vi "Main.vi"(10 "Number of socket":i32, 11 "Module Admin":refnum<class "Delacor_lib_QMH_Cloneable Module Admin.lvclass">) -> ()   [LabVIEW 2019, in "Test Unit.lvlib"]
doc: "This template is based off of the Queued Message Handler design pattern and the Queued Message Handler project template that ships with LabVIEW.\n\nThe main difference is that the queue is private to this module and communication between modules is performed via Broadcast and Request events.\n\nRequest events are wrapped in public API methods and are handled in the Event Handling Loop (EHL) of this VI. Any module can register for Broadcast events sent by this module. The EHL generates messages based on user interface actions.\n\nThe Message Handling Loop (MHL) processes messages generated by the EHL, or by other messages. The messages are string values, so new messages can be added easily to the Message Cases case structure in the MHL. Each message cluster can also provide an optional value for Message Data, which is a variant that can be converted to whatever message-specific data is required.\n_____\nBased on DQMH Project Template 7.0.1.1316."
uses:
  Test Unit.lvlib
  <vilib>/Delacor/Delacor QMH/Libraries/Cloneable Module Admin_class/Delacor_lib_QMH_Cloneable Module Admin.lvclass
  C:/Program Files (x86)/National Instruments/LabVIEW 2019/vi.lib/Delacor/Delacor QMH/Libraries/Module Admin_class/Delacor_lib_QMH_Module Admin.lvclass
  System.Windows.Forms
  <vilib>/Delacor/Delacor QMH/Libraries/Cloneable Module Admin_class/Delacor_lib_QMH_Cloneable Module Admin.lvclass/Delacor_lib_QMH_Cloneable Module Admin.ctl
  Module Data--cluster.ctl
  UUT Result.ctl
  <vilib>/Test Bench Framework/Test Executive.lvlibp/TestEngine/TestEngine/TestEngine/Typedefs/Report General.ctl
  <vilib>/Delacor/Delacor QMH/Libraries/Message Queue_class/Delacor_lib_QMH_Message Queue.lvclass/Delacor_lib_QMH_Message Queue.ctl
  Full User Interface/Send User Message Argument--cluster.ctl
  Stop Argument--cluster.ctl
  <vilib>/Delacor/Delacor QMH/Libraries/Module Admin_class/Delacor_lib_QMH_Module Admin.lvclass/Delacor_lib_QMH_Module Admin.ctl
  TitleWindows Argument--cluster.ctl
  Cofiguration Argument--cluster.ctl
  <vilib>/Test Bench Framework/Test Executive.lvlibp/TestEngine/TestEngine/TestEngine/Typedefs/TestEngine Cofiguration.ctl
  <vilib>/Test Bench Framework/Test Executive.lvlibp/TestEngine/TestEngine/TestEngine/Typedefs/Local Report Configuration.ctl
  <vilib>/Test Bench Framework/Test Executive.lvlibp/TestEngine/TestEngine/TestEngine/Report Format.ctl
  <vilib>/Test Bench Framework/Test Executive.lvlibp/TestEngine/TestEngine/TestEngine/Typedefs/Database Configuration.ctl
  Load Sequence Argument--cluster.ctl
  Write SN Argument--cluster.ctl
  UUT Test Argument--cluster.ctl
  UUTs Test Argument--cluster.ctl
  Terminate Test Argument--cluster.ctl
  Set Variable Argument--cluster.ctl
  Get Variable Argument--cluster.ctl
  Get Variable (Reply Payload)--cluster.ctl
  <vilib>/Delacor/Delacor QMH/Libraries/Message Queue_class/Delacor_lib_QMH_Enqueue Message (Single).vi
  <vilib>/Delacor/Delacor QMH/Libraries/Cloneable Module Admin_class/Delacor_lib_QMH_Get Module ID.vi
  <vilib>/Delacor/Delacor QMH/Libraries/Module Admin_class/Delacor_lib_QMH_Get External Launch.vi
  ffe5634f-0fac-49bb-99a4-0389974cdd12.vi
  <vilib>/Delacor/Delacor QMH/Libraries/Message Queue_class/Delacor_lib_QMH_Message Queue.lvclass
  <vilib>/Test Bench Framework/Test Executive(API).lvlib
  <vilib>/Test Bench Framework/Test Executive.lvlibp/TestEngine/TestEngine/TestEngine/Test Engine.lvclass
  Full User Interface/Full User Interface.lvlib
panel:
  in  "Panel":refnum<k24>(container)
  out "error out":errorcluster
  out "Status":string
  in  "Simulate EHL Error":bool
  in  "Simulate MHL Error":bool
  # "Other processes communicate with this Module via its Public API (wrappers for its Request Events).\n\nThis Module communicates with other processes via its Broadcast Events.\nAny process that wants to receive these messages can register for this module's Broadcast events."
  # "This template is for the DQMH framework. See the block diagram for more information on how to use this template."
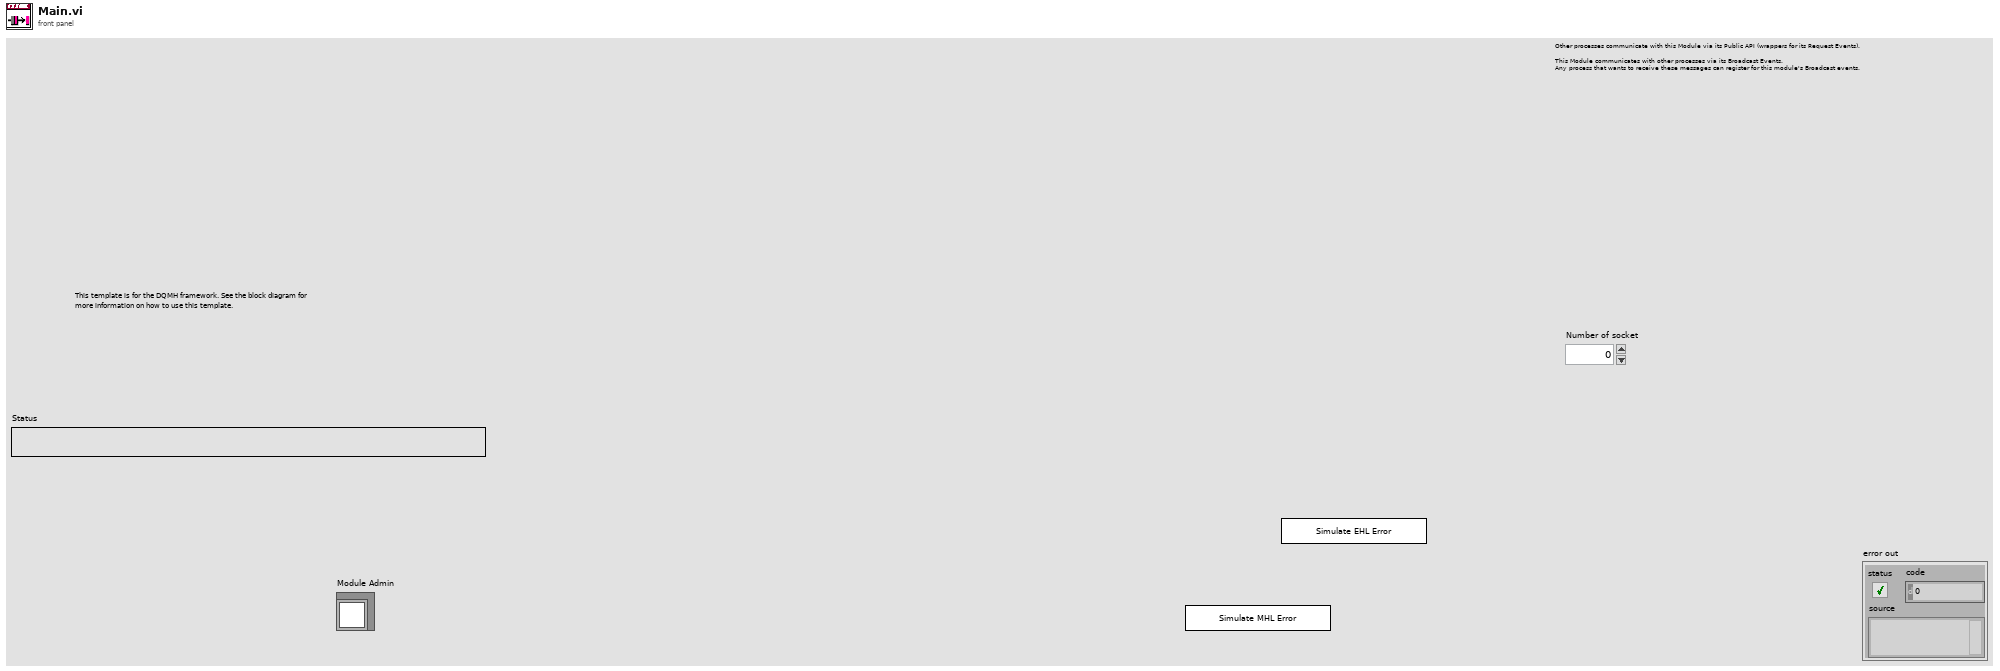
[diagram p1: front panel]
types:
  T1 = typedef "Test Unit.lvlib/Request Events--cluster.ctl" = cluster{"Stop Module":refnum<user-event>, "Show Panel":refnum<user-event>, "Hide Panel":refnum<user-event>, "Show Diagram":refnum<user-event>, "Get Module Execution Status":refnum<user-event>, "TileWindows":refnum<user-event>, "TitleWindows":refnum<user-event>, "Cofiguration":refnum<user-event>, "Load Sequence":refnum<user-event>, "Write SN":refnum<user-event>, "UUT Test":refnum<user-event>, "UUTs Test":refnum<user-event>, "Terminate Test":refnum<user-event>, "Set Variable":refnum<user-event>, "Get Variable":refnum<user-event>}
  T2 = cluster{"Event Registration Refnum":refnum<event-registration>, "Event Registration Refnum":refnum<event-registration>}
  T3 = typedef "Test Unit.lvlib/Module Data--cluster.ctl" = cluster{"Status":string, "exit":refnum<user-event>[], "UUT Result":map{i32, refnum<user-event>}}
  T4 = typedef "Test Unit.lvlib/UUT Result.ctl" = cluster{"Station":i32, "Socket":i32, "DetailTestResult":string[][], "Report Path":path, "General":T5}
  T5 = typedef "Test Executive.lvlibp/Test Engine.lvlib/Test Engine.lvclass/Report General.ctl" = cluster{"Sequence Path":path, "Serial Number":string, "Test Date Time":timestamp, "UUT Status":string, "Faulty Item":string, "Seconds Executing":dbl}
  T6 = typedef "Full User Interface.lvlib/Send User Message Argument--cluster.ctl" = cluster{"Station ID":i32, "Socket":i32, "UserMessage":string, "MessageData":variant}
  T7 = enum32{"invalid lock state", "Not Locked", "Locked (No Password)", "Password-protected"}
  T8 = typedef "Test Unit.lvlib/Stop Argument--cluster.ctl" = cluster{"Module ID":i32, "Origin":string, "Exit via Stop Module Req?":bool, "Wait for Module to stop?":bool}
  T9 = typedef "Test Unit.lvlib/TitleWindows Argument--cluster.ctl" = cluster{"Module ID":i32, "TitleWindows":bool, "dont initi":bool}
  T10 = typedef "Test Unit.lvlib/Cofiguration Argument--cluster.ctl" = cluster{"Module ID":i32, "TestEngine Cofiguration":T11}
  T11 = typedef "Test Executive.lvlibp/Test Engine.lvlib/Test Engine.lvclass/TestEngine Cofiguration.ctl" = cluster{"Break on Failure":bool, "Automatically handle TestVI error":cluster{"Enable":bool, "Handle":enum16{"Termination test", "Ignore error"}}, "Local Report Configuration":T12, "Database Configuration":T14, "Ignore breakpoint":bool, "Filter Result":bool}
  T12 = typedef "Test Executive.lvlibp/Test Engine.lvlib/Test Engine.lvclass/Local Report Configuration.ctl" = cluster{"Report Folder Path":path, "Format":T13, "Disable":bool, "Build Date Folder?":bool}
  T13 = typedef "Test Executive.lvlibp/Test Engine.lvlib/Test Engine.lvclass/Report Format.ctl" = enum16{"Excel", "CSV(Tab)", "CSV(,)", "CSV(;)", "TEXT", "HTML"}
  T14 = typedef "Test Executive.lvlibp/Test Engine.lvlib/Test Engine.lvclass/Database Configuration.ctl" = cluster{"Connection String Expression":string, "Microsoft Data Link File":path, "Connection Type":enum16{"Use Connection String Expression", "Use Microsoft Data Link File"}, "Enable":bool}
  T15 = typedef "Test Unit.lvlib/Load Sequence Argument--cluster.ctl" = cluster{"Module ID":i32, "File Pathname":path, "Sequence":string}
  T16 = typedef "Test Unit.lvlib/Write SN Argument--cluster.ctl" = cluster{"Module ID":i32, "Socket":i32, "Serial Number":string}
  T17 = typedef "Test Unit.lvlib/UUT Test Argument--cluster.ctl" = cluster{"Module ID":i32, "Socket":i32}
  T18 = typedef "Test Unit.lvlib/UUTs Test Argument--cluster.ctl" = cluster{"Module ID":i32, "Enable Socket":bool[]}
  T19 = typedef "Test Unit.lvlib/Terminate Test Argument--cluster.ctl" = cluster{"Module ID":i32, "Abort VI":bool}
  T20 = typedef "Test Unit.lvlib/Set Variable Argument--cluster.ctl" = cluster{"Module ID":i32, "Variable":string, "Socket":i32, "Value":variant}
  T21 = typedef "Test Unit.lvlib/Get Variable Argument--cluster.ctl" = cluster{"Module ID":i32, "Socket":i32, "Variable":string, "Wait Notifier":refnum<notifier>, "wait for reply":bool}
  T22 = enum32{"Invalid", "Standard", "Closed", "Hidden", "Minimized", "Maximized"}
  T23 = typedef "Test Unit.lvlib/Get Variable (Reply Payload)--cluster.ctl" = cluster{"Module ID":i32, "Value":variant, "Variable not found?":bool, "timed out?":bool, "error":errorcluster}
  T24 = cluster{"Left":i32, "Top":i32, "Right":i32, "Bottom":i32}
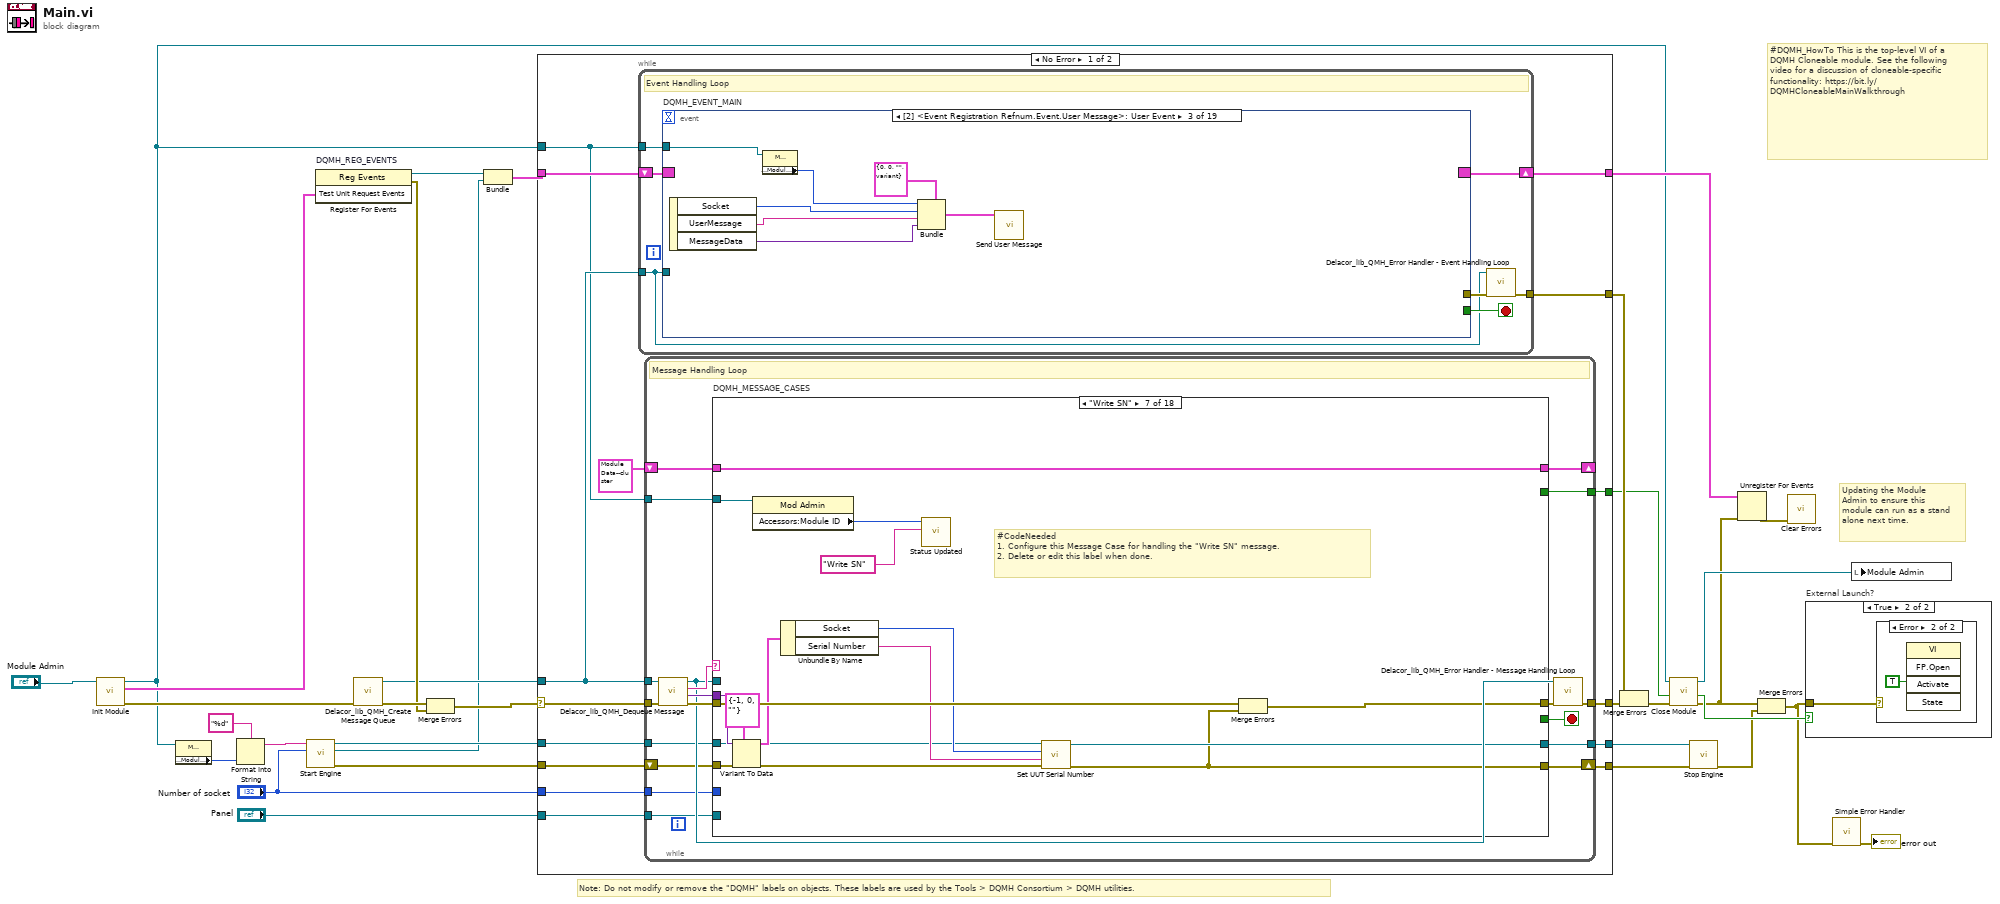
[diagram p0: block diagram]
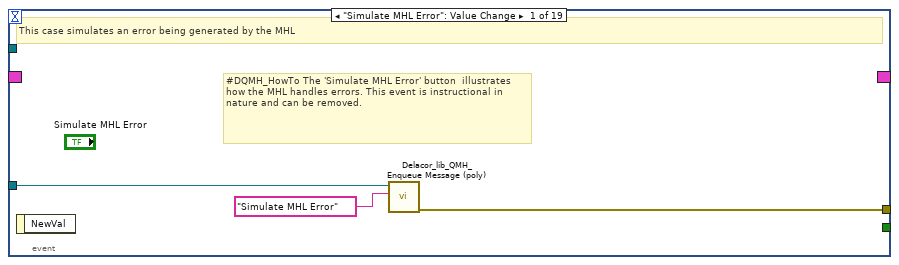
[diagram p2: hidden frame]
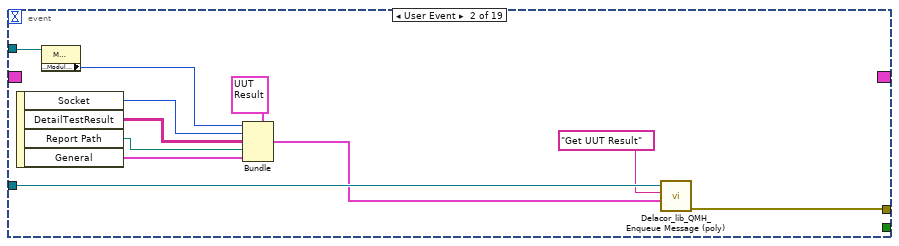
[diagram p3: hidden frame]
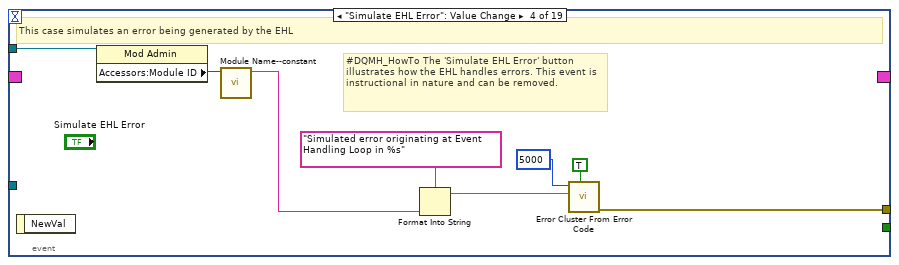
[diagram p4: hidden frame]
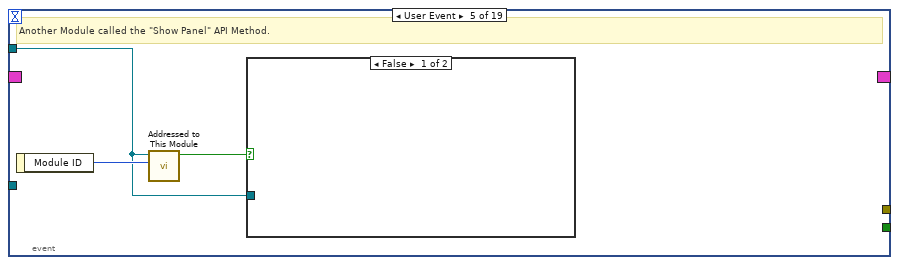
[diagram p5: hidden frame]
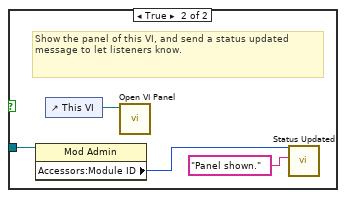
[diagram p6: hidden frame]
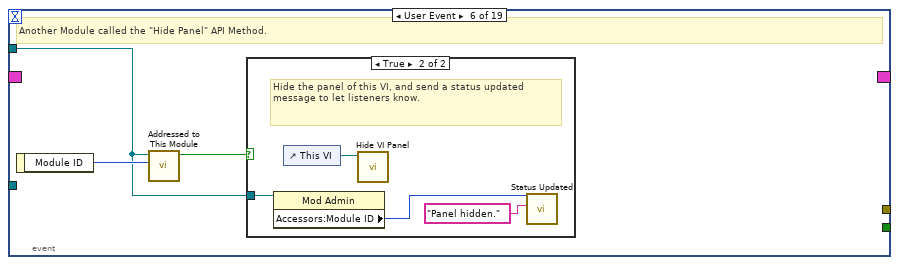
[diagram p7: hidden frame]
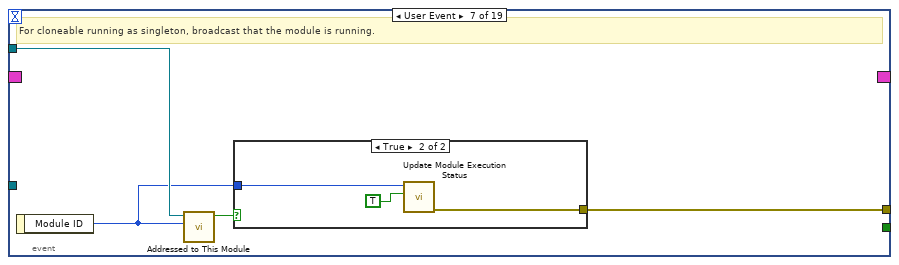
[diagram p9: hidden frame]
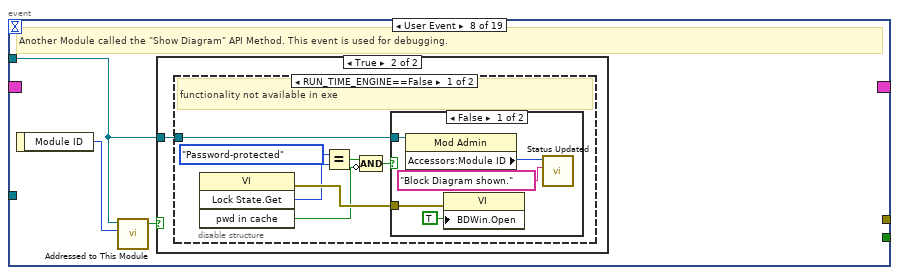
[diagram p11: hidden frame]
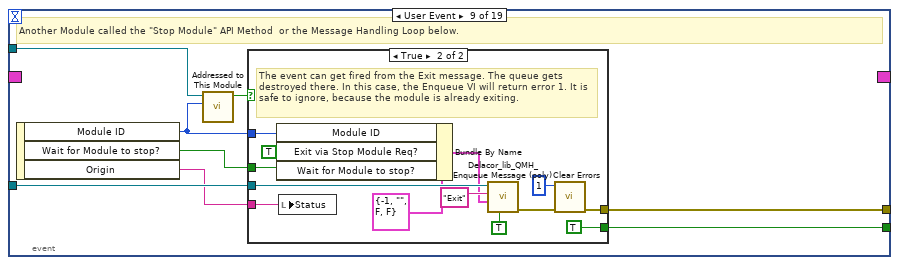
[diagram p15: hidden frame]
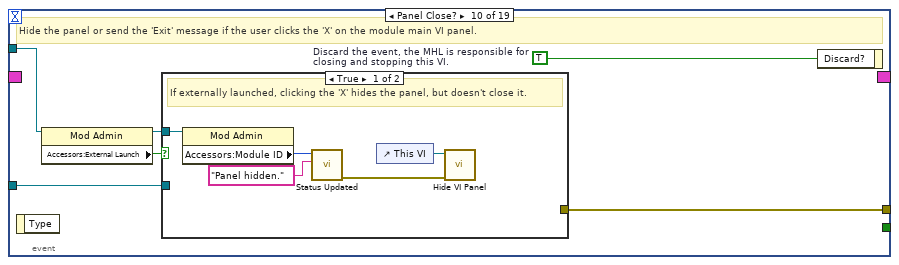
[diagram p17: hidden frame]
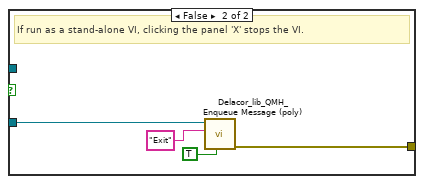
[diagram p18: hidden frame]
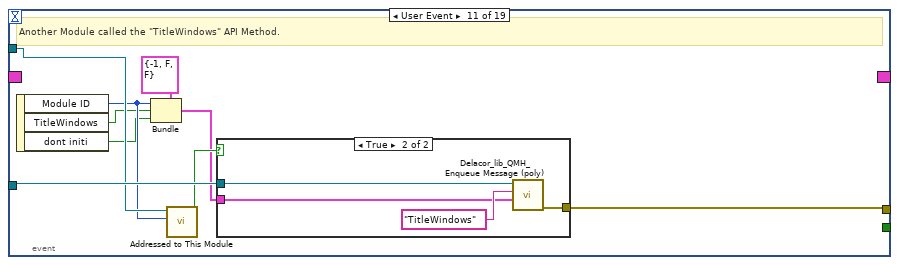
[diagram p19: hidden frame]
diagram:
  # "#DQMH_HowTo This is the top-level VI of a DQMH Cloneable module. See the following video for a discussion of cloneable-specific functionality: https://bit.ly/DQMHCloneableMainWalkthrough"
  # "Note: Do not modify or remove the \"DQMH\" labels on objects. These labels are used by the Tools > DQMH Consortium > DQMH utilities."
  # "Updating the Module Admin to ensure this module can run as a stand alone next time."
  n1 = call "Init Module.vi"("Cloneable Module Admin in"="Module Admin") -> ("error out"=w29:errorcluster, "Test Unit Request Events"=w24:T1, "Cloneable Module Admin out"=w17:refnum<class "Delacor_lib_QMH_Cloneable Module Admin.lvclass">)  [unwired: 8 in]
  n2 = property class="Mod Admin"(reference=w17) -> ("Accessors:Module ID"=w16:i32)  [unwired: 1 in, 2 out]
  n3 = Format Into String(format string="%d", w16) -> (resulting string=w14:string)  [unwired: 2 in, 1 out]
  n4 = call <vilib>:"Start Engine.vi"("Number of Socket"="Number of socket", "Process"=w14) -> ("error out"=w19:errorcluster, "Event Registration Refnum"=w3:refnum<event-registration>, "Test Executive Manage out"=w18:refnum<class "Test Executive Manage.lvclass">)  [unwired: 7 in]
  n5 = register-events "DQMH_REG_EVENTS"(w24) -> (reference out=w25:refnum<event-registration>, error out=w27:errorcluster)  [unwired: 2 in]
  n6 = call <vilib>:"Delacor_lib_QMH_Create Message Queue.vi"("error in"=w29) -> ("error out"=w28:errorcluster, "Message Queue"=w10:refnum<class "Delacor_lib_QMH_Message Queue.lvclass">)  [unwired: 9 in]
  n7 = Merge Errors(w28, w27) -> (w9:errorcluster)
  n8 = Bundle("Event Registration Refnum"=w25, "Event Registration Refnum"=w3) -> (w4:T2)  [unwired: 1 in]
  n9 = case shown="No Error" w9 {
    selector: w9 -> [w45 w611]
    tunnel: [w47 w610] -> w30
    tunnel: [w44 w609] -> w26
    tunnel: w4 -> [w42 w609]
    tunnel: w10 -> [w41 w602]
    tunnel: [w46 _] -> w31
    tunnel: w17 -> [w40 w605]
    tunnel: [w39 _] -> w21
    tunnel: w19 -> [w38 w600]
    tunnel: w18 -> [w37 w601]
    tunnel: [w36 w601] -> w13
    tunnel: [w35 w600] -> w12
    tunnel: "Number of socket" -> [w34 _]
    tunnel: "Panel" -> [w33 _]
    frame No Error {
      n10 = while {
        tunnel: w41 -> [w48]
        shift-right: [w51] -> w44
        shift-left: w42 -> [w52]
        tunnel: [w53] -> w46
        tunnel: w40 -> [w49]
        stop <- w50 stop-if-true
        # "Event Handling Loop"
        n11 = event "DQMH_EVENT_MAIN" shown="[2] <Event Registration Refnum.Event.User Message>: User Event" {
          selector: w52 -> [_ _ _ _ _ _ _ _ _ _ _ _ _ _ _ _ _ _ _]
          dyn-events: [_ _ _ _ _ _ _ _ _ _ _ _ _ _ _ _ _ _ _] -> w51
          timeout: _ -> [_ _ _ _ _ _ _ _ _ _ _ _ _ _ _ _ _ _ _]
          tunnel: [_ _ _ _ _ _ _ _ w124 _ _ _ _ _ _ _ _ _ _] -> w50
          tunnel: w48 -> [w56 w68 _ _ _ _ _ _ w127 w144 w165 w177 w190 w203 w215 w227 w239 w253 w268]
          tunnel: [w57 w66 _ w83 _ _ w101 _ w128 w147 w158 w170 w182 w195 w208 w220 w232 w244 w258] -> w54
          tunnel: w49 -> [_ w63 w75 w82 w84 w91 w99 w105 w126 w145 w163 w175 w188 w201 w213 w225 w237 w251 w266]
          event "Simulate MHL Error": Value Change {
            # "#DQMH_HowTo The 'Simulate MHL Error' button  illustrates how the MHL handles errors. This event is instructional in nature and can be removed."
            # "This case simulates an error being generated by the MHL"
            n12 = event-data() -> ()  [unwired: 1 in, 1 out]
            n13 = call-poly <vilib>:"Delacor_lib_QMH_Enqueue Message (poly).vi"("Message"="Simulate MHL Error", "Message Queue in"=w56) -> ("error out"=w57:errorcluster)  [unwired: 8 in, 1 out]
          }
          event User Event {
            n14 = event-data() -> ("Socket"=w61:i32, "DetailTestResult"=w60:string[][], "Report Path"=w59:path, "General"=w58:T5)  [unwired: 1 in]
            n15 = property class="Mod Admin"(reference=w63) -> ("Accessors:Module ID"=w62:i32)  [unwired: 1 in, 2 out]
            n16 = Bundle(cluster=T4 {"Station"=0, "Socket"=0, "DetailTestResult"=[], "Report Path"=path "", "General"={"Sequence Path"=path "", "Serial Number"="", "Test Date Time"=timestamp(0 s since 1904-01-01), "UUT Status"="", "Faulty Item"="", "Seconds Executing"=0.0}} ("output cluster"), "Station"=w62, "Socket"=w61, "DetailTestResult"=w60, "Report Path"=w59, "General"=w58) -> (w67:T4)
            n17 = call-poly <vilib>:"Delacor_lib_QMH_Enqueue Message (poly).vi"("Message Data"=w67, "Message"="Get UUT Result", "Message Queue in"=w68) -> ("error out"=w66:errorcluster)  [unwired: 7 in, 1 out]
          }
          event User Event {
            n18 = event-data() -> ("Socket"=w72:i32, "UserMessage"=w71:string, "MessageData"=w70:variant)  [unwired: 1 in]
            n19 = property class="Mod Admin"(reference=w75) -> ("Accessors:Module ID"=w73:i32)  [unwired: 1 in, 2 out]
            n20 = Bundle(cluster=T6 {"Station ID"=0, "Socket"=0, "UserMessage"="", "MessageData"=variant(cluster{"Socket":i32, "UserMessage":string, "MessageData":variant} {"Socket"=0, "UserMessage"="", "MessageData"=variant})} ("DQMH_ARG"), "Station ID"=w73, "Socket"=w72, "UserMessage"=w71, "MessageData"=w70) -> (w69:T6)
            n21 = call "Send User Message.vi"("DQMH_ARG"=w69) -> ()  [unwired: 10 in, 1 out]
          }
          event "Simulate EHL Error": Value Change {
            # "#DQMH_HowTo The 'Simulate EHL Error' button  illustrates how the EHL handles errors. This event is instructional in nature and can be removed."
            # "This case simulates an error being generated by the EHL"
            n22 = event-data() -> ()  [unwired: 1 in, 1 out]
            n23 = property on="Property Node" class="Mod Admin"(reference=w82) -> ("Accessors:Module ID"=w81:i32)  [unwired: 1 in, 2 out]
            n24 = call "Module Name--constant.vi"("Module ID"=w81) -> ("Module Name"=w76:string)  [unwired: 10 in]
            n25 = Format Into String(format string="Simulated error originating at Event Handling Loop in %s", w76) -> (resulting string=w79:string)  [unwired: 2 in, 1 out]
            n26 = call <vilib>:"Error Cluster From Error Code.vi"("show call chain? (False)"=TRUE, "error message (\"\")"=w79, "error code (0)"=5000) -> ("error out"=w83:errorcluster)  [unwired: 6 in]
          }
          event User Event {
            # "Another Module called the \"Show Panel\" API Method."
            n27 = event-data() -> ("Module ID"=w85:i32)  [unwired: 1 in]
            n28 = call "Addressed to This Module.vi"("Module ID from Argument"=w85, "Module Admin"=w84) -> ("Addressed to this instance?"=w86:bool)  [unwired: 8 in, 1 out]
            n29 = case shown="False" w86 {
              tunnel: w84 -> [_ w88]
              frame False {
              }
              frame True {
                # "Show the panel of this VI, and send a status updated message to let listeners know."
                n30 = property on="Property Node" class="Mod Admin"(reference=w88) -> ("Accessors:Module ID"=w87:i32)  [unwired: 1 in, 2 out]
                n31 = control-ref of="This VI"() -> (w90:refnum<vi>)
                n32 = call "Open VI Panel.vi"("VI"=w90) -> ()  [unwired: 10 in, 1 out]
                n33 = call "Status Updated.vi"("Status"="Panel shown." ("format string"), "Module ID"=w87) -> ()  [unwired: 9 in, 1 out]
              }
            }
          }
          event User Event {
            # "Another Module called the \"Hide Panel\" API Method."
            n34 = event-data() -> ("Module ID"=w92:i32)  [unwired: 1 in]
            n35 = call "Addressed to This Module.vi"("Module ID from Argument"=w92, "Module Admin"=w91) -> ("Addressed to this instance?"=w93:bool)  [unwired: 8 in, 1 out]
            n36 = case shown="True" w93 {
              tunnel: w91 -> [_ w95]
              frame False {
              }
              frame True {
                # "Hide the panel of this VI, and send a status updated message to let listeners know."
                n37 = property on="Property Node" class="Mod Admin"(reference=w95) -> ("Accessors:Module ID"=w94:i32)  [unwired: 1 in, 2 out]
                n38 = control-ref of="This VI"() -> (w97:refnum<vi>)
                n39 = call "Hide VI Panel.vi"("VI"=w97) -> ()  [unwired: 10 in, 1 out]
                n40 = call "Status Updated.vi"("Status"="Panel hidden." ("format string"), "Module ID"=w94) -> ()  [unwired: 9 in, 1 out]
              }
            }
          }
          event User Event {
            # "For cloneable running as singleton, broadcast that the module is running."
            n41 = event-data() -> ("Module ID"=w98:i32)  [unwired: 1 in]
            n42 = call "Addressed to This Module.vi"("Module ID from Argument"=w98, "Module Admin"=w99) -> ("Addressed to this instance?"=w100:bool)  [unwired: 8 in, 1 out]
            n43 = case shown="True" w100 {
              tunnel: [_ w104] -> w101
              tunnel: w98 -> [_ w103]
              frame False {
              }
              frame True {
                n44 = call "Update Module Execution Status.vi"("Running?"=TRUE, "Module ID"=w103) -> ("error out"=w104:errorcluster)  [unwired: 9 in]
              }
            }
          }
          event User Event {
            # "Another Module called the \"Show Diagram\" API Method. This event is used for debugging."
            n45 = event-data() -> ("Module ID"=w106:i32)  [unwired: 1 in]
            n46 = call "Addressed to This Module.vi"("Module ID from Argument"=w106, "Module Admin"=w105) -> ("Addressed to this instance?"=w107:bool)  [unwired: 8 in, 1 out]
            n47 = case shown="True" w107 {
              tunnel: w105 -> [_ w108]
              frame False {
              }
              frame True {
                n48 = disable-structure shown="RUN_TIME_ENGINE==False" {
                  disable-tunnel: w108 -> [w109 _]
                  frame condition #0 (active) {
                    # "functionality not available in exe"
                    n49 = invoke on="Invoke Node" class="VI" method="Lock State.Get"() -> (error out=w115:errorcluster, "Get Lock State"=w114:T7, "pwd in cache"=w111:bool)  [unwired: 4 in, 1 out]
                    n50 = Equal?(x=T7."Password-protected", y=w114) -> (x = y?=w112:bool)
                    n51 = Compound Arithmetic op=AND(w112, invert w111) -> (w110:bool)
                    n52 = case shown="False" w110 {
                      tunnel: w115 -> [w120 _]
                      tunnel: w109 -> [w117 _]
                      frame False {
                        n53 = property on="Property Node" class="Mod Admin"(reference=w117) -> ("Accessors:Module ID"=w116:i32)  [unwired: 1 in, 2 out]
                        n54 = property on="Property Node" class="VI"(error in=w120, "BDWin.Open"=TRUE ("Block Diagram Window:Open")) -> ()  [unwired: 1 in, 2 out]
                        n55 = call "Status Updated.vi"("Status"="Block Diagram shown." ("format string"), "Module ID"=w116) -> ()  [unwired: 9 in, 1 out]
                      }
                      frame True {
                        # "Password-protected VI, and the password is not in the cache. Do not show the diagram."
                      }
                    }
                  }
                  frame condition #1 {
                  }
                }
              }
            }
          }
          event User Event {
            # "Another Module called the \"Stop Module\" API Method  or the Message Handling Loop below."
            n56 = event-data() -> ("Module ID"=w122:i32, "Wait for Module to stop?"=w123:bool, "Origin"=w121:string)  [unwired: 1 in]
            n57 = call "Addressed to This Module.vi"("Module ID from Argument"=w122, "Module Admin"=w126) -> ("Addressed to this instance?"=w125:bool)  [unwired: 8 in, 1 out]
            n58 = case shown="True" w125 {
              tunnel: [_ w140] -> w128
              tunnel: w127 -> [_ w136]
              tunnel: [_ TRUE] -> w124
              tunnel: w123 -> [_ w131]
              tunnel: w122 -> [_ w133]
              tunnel: w121 -> [_ w129]
              frame False {
              }
              frame True {
                # "The event can get fired from the Exit message. The queue gets destroyed there. In this case, the Enqueue VI will return error 1. It is safe to ignore, because the module is already exiting."
                n59 = Bundle By Name(cluster=T8 {"Module ID"=-1, "Origin"="", "Exit via Stop Module Req?"=FALSE, "Wait for Module to stop?"=FALSE} ("Stop Argument"), "Module ID"=w133, "Exit via Stop Module Req?"=TRUE, "Wait for Module to stop?"=w131) -> (w130:T8)
                n60 = local write "Status"(w129) -> ()
                n61 = call-poly <vilib>:"Delacor_lib_QMH_Enqueue Message (poly).vi"("Priority Message? (F)"=TRUE, "Message Data"=w130, "Message"="Exit", "Message Queue in"=w136) -> ("error out"=w141:errorcluster)  [unwired: 6 in, 1 out]
                n62 = call <vilib>:"Clear Errors.vi"("error in (no error)"=w141, "specific error code to clear (0: all)"=1) -> ("error out"=w140:errorcluster)  [unwired: 4 in, 1 out]
              }
            }
          }
          event Panel Close? {
            w146 = TRUE  # Discard the event, the MHL is responsible for closing and stopping this VI.
            # "Hide the panel or send the 'Exit' message if the user clicks the 'X' on the module main VI panel."
            n63 = event-data() -> ()  [unwired: 1 in, 1 out]
            n64 = property on="Property Node" class="Mod Admin"(reference=w145) -> (reference out=w142:refnum<class "Delacor_lib_QMH_Cloneable Module Admin.lvclass">, "Accessors:External Launch"=w143:bool)  [unwired: 1 in, 1 out]
            n65 = case shown="True" w143 {
              tunnel: w144 -> [_ w155]
              tunnel: [_ w156] -> w147
              tunnel: w142 -> [w150 _]
              frame True {
                # "If externally launched, clicking the 'X' hides the panel, but doesn't close it."
                n66 = property on="Property Node" class="Mod Admin"(reference=w150) -> ("Accessors:Module ID"=w149:i32)  [unwired: 1 in, 2 out]
                n67 = call "Status Updated.vi"("Status"="Panel hidden." ("format string"), "Module ID"=w149) -> ("error out"=w148:errorcluster)  [unwired: 9 in]
                n68 = control-ref of="This VI"() -> (w152:refnum<vi>)
                n69 = call "Hide VI Panel.vi"("error in"=w148, "VI"=w152) -> ()  [unwired: 9 in, 1 out]
              }
              frame False {
                # "If run as a stand-alone VI, clicking the panel 'X' stops the VI."
                n70 = call-poly <vilib>:"Delacor_lib_QMH_Enqueue Message (poly).vi"("Priority Message? (F)"=TRUE, "Message"="Exit", "Message Queue in"=w155) -> ("error out"=w156:errorcluster)  [unwired: 7 in, 1 out]
              }
            }
            n71 = event-data ("Event Filter Node")("Discard?"=w146) -> ()  [unwired: 1 in, 1 out]
          }
          event User Event {
            # "Another Module called the \"TitleWindows\" API Method."
            n72 = event-data() -> ("Module ID"=w160:i32, "TitleWindows"=w159:bool, "dont initi"=w157:bool)  [unwired: 1 in]
            n73 = Bundle(cluster=T9 {"Module ID"=-1, "TitleWindows"=FALSE, "dont initi"=FALSE} ("TitleWindows Argument"), "Module ID"=w160, "TitleWindows"=w159, "dont initi"=w157) -> (w161:T9)
            n74 = call "Addressed to This Module.vi"("Module ID from Argument"=w160, "Module Admin"=w163) -> ("Addressed to this instance?"=w164:bool)  [unwired: 8 in, 1 out]
            n75 = case shown="True" w164 {
              tunnel: w165 -> [_ w169]
              tunnel: w161 -> [_ w167]
              tunnel: [_ w166] -> w158
              frame False {
              }
              frame True {
                n76 = call-poly <vilib>:"Delacor_lib_QMH_Enqueue Message (poly).vi"("Message Data"=w167, "Message"="TitleWindows", "Message Queue in"=w169) -> ("error out"=w166:errorcluster)  [unwired: 7 in, 1 out]
              }
            }
          }
          event User Event {
            # "Another Module called the \"Cofiguration\" API Method."
            n77 = event-data() -> ("Module ID"=w172:i32, "TestEngine Cofiguration"=w171:T11)  [unwired: 1 in]
            n78 = Bundle(cluster=T10 {"Module ID"=-1, "TestEngine Cofiguration"={"Break on Failure"=FALSE, "Automatically handle TestVI error"={"Enable"=FALSE, "Handle"=enum."Termination test"}, "Local Report Configuration"={"Report Folder Path"=path "", "Format"=enum."Excel", "Disable"=FALSE, "Build Date Folder?"=FALSE}, "Database Configuration"={"Connection String Expression"="", "Microsoft Data Link File"=path "", "Connection Type"=enum."Use Connection String Expression", "Enable"=FALSE}, "Ignore breakpoint"=FALSE, "Filter Result"=FALSE}} ("Cofiguration Argument"), "Module ID"=w172, "TestEngine Cofiguration"=w171) -> (w173:T10)
            n79 = call "Addressed to This Module.vi"("Module ID from Argument"=w172, "Module Admin"=w175) -> ("Addressed to this instance?"=w176:bool)  [unwired: 8 in, 1 out]
            n80 = case shown="True" w176 {
              tunnel: w177 -> [_ w181]
              tunnel: w173 -> [_ w179]
              tunnel: [_ w178] -> w170
              frame False {
              }
              frame True {
                n81 = call-poly <vilib>:"Delacor_lib_QMH_Enqueue Message (poly).vi"("Message Data"=w179, "Message"="Cofiguration", "Message Queue in"=w181) -> ("error out"=w178:errorcluster)  [unwired: 7 in, 1 out]
              }
            }
          }
          event User Event {
            # "Another Module called the \"Load Sequence\" API Method."
            n82 = event-data() -> ("Module ID"=w185:i32, "File Pathname"=w184:path, "Sequence"=w183:string)  [unwired: 1 in]
            n83 = Bundle(cluster=T15 {"Module ID"=-1, "File Pathname"=path "", "Sequence"="Main_Sequence"} ("Load Sequence Argument"), "Module ID"=w185, "File Pathname"=w184, "Sequence"=w183) -> (w186:T15)
            n84 = call "Addressed to This Module.vi"("Module ID from Argument"=w185, "Module Admin"=w188) -> ("Addressed to this instance?"=w189:bool)  [unwired: 8 in, 1 out]
            n85 = case shown="True" w189 {
              tunnel: w190 -> [_ w194]
              tunnel: w186 -> [_ w192]
              tunnel: [_ w191] -> w182
              frame False {
              }
              frame True {
                n86 = call-poly <vilib>:"Delacor_lib_QMH_Enqueue Message (poly).vi"("Message Data"=w192, "Message"="Load Sequence", "Message Queue in"=w194) -> ("error out"=w191:errorcluster)  [unwired: 7 in, 1 out]
              }
            }
          }
          event User Event {
            # "Another Module called the \"Write SN\" API Method."
            n87 = event-data() -> ("Module ID"=w198:i32, "Socket"=w197:i32, "Serial Number"=w196:string)  [unwired: 1 in]
            n88 = Bundle(cluster=T16 {"Module ID"=-1, "Socket"=0, "Serial Number"=""} ("Write SN Argument"), "Module ID"=w198, "Socket"=w197, "Serial Number"=w196) -> (w199:T16)
            n89 = call "Addressed to This Module.vi"("Module ID from Argument"=w198, "Module Admin"=w201) -> ("Addressed to this instance?"=w202:bool)  [unwired: 8 in, 1 out]
            n90 = case shown="True" w202 {
              tunnel: w203 -> [_ w207]
              tunnel: w199 -> [_ w205]
              tunnel: [_ w204] -> w195
              frame False {
              }
              frame True {
                n91 = call-poly <vilib>:"Delacor_lib_QMH_Enqueue Message (poly).vi"("Message Data"=w205, "Message"="Write SN", "Message Queue in"=w207) -> ("error out"=w204:errorcluster)  [unwired: 7 in, 1 out]
              }
            }
          }
          event User Event {
            # "Another Module called the \"UUT Test\" API Method."
            n92 = event-data() -> ("Module ID"=w210:i32, "Socket"=w209:i32)  [unwired: 1 in]
            n93 = Bundle(cluster=T17 {"Module ID"=-1, "Socket"=0} ("UUT Test Argument"), "Module ID"=w210, "Socket"=w209) -> (w211:T17)
            n94 = call "Addressed to This Module.vi"("Module ID from Argument"=w210, "Module Admin"=w213) -> ("Addressed to this instance?"=w214:bool)  [unwired: 8 in, 1 out]
            n95 = case shown="True" w214 {
              tunnel: w215 -> [_ w219]
              tunnel: w211 -> [_ w217]
              tunnel: [_ w216] -> w208
              frame False {
              }
              frame True {
                n96 = call-poly <vilib>:"Delacor_lib_QMH_Enqueue Message (poly).vi"("Message Data"=w217, "Message"="UUT Test", "Message Queue in"=w219) -> ("error out"=w216:errorcluster)  [unwired: 7 in, 1 out]
              }
            }
          }
          event User Event {
            # "Another Module called the \"UUTs Test\" API Method."
            n97 = event-data() -> ("Module ID"=w222:i32, "Enable Socket"=w221:bool[])  [unwired: 1 in]
            n98 = Bundle(cluster=T18 {"Module ID"=-1, "Enable Socket"=[]} ("UUTs Test Argument"), "Module ID"=w222, "Enable Socket"=w221) -> (w223:T18)
            n99 = call "Addressed to This Module.vi"("Module ID from Argument"=w222, "Module Admin"=w225) -> ("Addressed to this instance?"=w226:bool)  [unwired: 8 in, 1 out]
            n100 = case shown="True" w226 {
              tunnel: w227 -> [_ w231]
              tunnel: w223 -> [_ w229]
              tunnel: [_ w228] -> w220
              frame False {
              }
              frame True {
                n101 = call-poly <vilib>:"Delacor_lib_QMH_Enqueue Message (poly).vi"("Message Data"=w229, "Message"="UUTs Test", "Message Queue in"=w231) -> ("error out"=w228:errorcluster)  [unwired: 7 in, 1 out]
              }
            }
          }
          event User Event {
            # "Another Module called the \"Terminate Test\" API Method."
            n102 = event-data() -> ("Module ID"=w234:i32, "Abort VI"=w233:bool)  [unwired: 1 in]
            n103 = Bundle(cluster=T19 {"Module ID"=-1, "Abort VI"=FALSE} ("Terminate Test Argument"), "Module ID"=w234, "Abort VI"=w233) -> (w235:T19)
            n104 = call "Addressed to This Module.vi"("Module ID from Argument"=w234, "Module Admin"=w237) -> ("Addressed to this instance?"=w238:bool)  [unwired: 8 in, 1 out]
            n105 = case shown="True" w238 {
              tunnel: w239 -> [_ w243]
              tunnel: w235 -> [_ w241]
              tunnel: [_ w240] -> w232
              frame False {
              }
              frame True {
                n106 = call-poly <vilib>:"Delacor_lib_QMH_Enqueue Message (poly).vi"("Message Data"=w241, "Message"="Terminate Test", "Message Queue in"=w243) -> ("error out"=w240:errorcluster)  [unwired: 7 in, 1 out]
              }
            }
          }
          event User Event {
            # "Another Module called the \"Set Variable\" API Method."
            n107 = event-data() -> ("Module ID"=w248:i32, "Variable"=w247:string, "Socket"=w246:i32, "Value"=w245:variant)  [unwired: 1 in]
            n108 = Bundle(cluster=T20 {"Module ID"=-1, "Variable"="", "Socket"=0, "Value"=variant} ("Set Variable Argument"), "Module ID"=w248, "Variable"=w247, "Socket"=w246, "Value"=w245) -> (w249:T20)
            n109 = call "Addressed to This Module.vi"("Module ID from Argument"=w248, "Module Admin"=w251) -> ("Addressed to this instance?"=w252:bool)  [unwired: 8 in, 1 out]
            n110 = case shown="True" w252 {
              tunnel: w253 -> [_ w257]
              tunnel: w249 -> [_ w255]
              tunnel: [_ w254] -> w244
              frame False {
              }
              frame True {
                n111 = call-poly <vilib>:"Delacor_lib_QMH_Enqueue Message (poly).vi"("Message Data"=w255, "Message"="Set Variable", "Message Queue in"=w257) -> ("error out"=w254:errorcluster)  [unwired: 7 in, 1 out]
              }
            }
          }
          event User Event {
            # "Another Module called the \"Get Variable\" API Method."
            n112 = event-data() -> ("Module ID"=w263:i32, "Socket"=w262:i32, "Variable"=w261:string, "Wait Notifier"=w260:refnum<notifier>, "wait for reply"=w259:bool)  [unwired: 1 in]
            n113 = Bundle(cluster=T21 {"Module ID"=-1, "Socket"=0, "Variable"="", "Wait Notifier"=refnum, "wait for reply"=FALSE} ("Get Variable Argument"), "Module ID"=w263, "Socket"=w262, "Variable"=w261, "Wait Notifier"=w260, "wait for reply"=w259) -> (w264:T21)
            n114 = call "Addressed to This Module.vi"("Module ID from Argument"=w263, "Module Admin"=w266) -> ("Addressed to this instance?"=w267:bool)  [unwired: 8 in, 1 out]
            n115 = case shown="True" w267 {
              tunnel: w268 -> [_ w272]
              tunnel: w264 -> [_ w270]
              tunnel: [_ w269] -> w258
              frame False {
              }
              frame True {
                n116 = call-poly <vilib>:"Delacor_lib_QMH_Enqueue Message (poly).vi"("Message Data"=w270, "Message"="Get Variable", "Message Queue in"=w272) -> ("error out"=w269:errorcluster)  [unwired: 7 in, 1 out]
              }
            }
          }
        }
        n117 = call-dynamic "Delacor_lib_QMH_Error Handler - Event Handling Loop.vi"("error in"=w54, "Message Queue in"=w48) -> ("dup error in"=w53:errorcluster)  [unwired: 8 in, 1 out]
      }
      n118 = while {
        tunnel: w41 -> [w279]
        shift-right: [w286] -> _
        shift-left: T3 {"Status"="", "exit"=[], "UUT Result"={}} ("Data Cluster") -> [w287]
        tunnel: w45 -> [w290]
        tunnel: [w288] -> w47
        tunnel: w40 -> [w281]
        tunnel: [w280] -> w39
        tunnel: w37 -> [w277]
        tunnel: [w276] -> w36
        shift-right: [w275] -> w35
        shift-left: w38 -> [w278]
        tunnel: w34 -> [w274]
        tunnel: w33 -> [w273]
        stop <- w285 stop-if-true
        # "Message Handling Loop"
        n119 = call-dynamic "Delacor_lib_QMH_Dequeue Message.vi"("error in"=w290, "Message Queue in"=w279) -> ("error out"=w289:errorcluster, "Message Data"=w283:variant, "Message"=w284:string, "Message Queue out"=w282:refnum<class "Delacor_lib_QMH_Message Queue.lvclass">)  [unwired: 6 in]
        n120 = case "DQMH_MESSAGE_CASES" shown="\"Write SN\"" w284 {
          selector: w284 -> [_ _ _ _ _ _ _ _ _ _ _ _ _ _ _ _ _ w589]
          tunnel: w282 -> [w298 _ _ w356 _ _ _ _ _ _ _ _ _ _ w535 _ w577 _]
          tunnel: w289 -> [w315 w321 w327 w355 w376 w400 w416 w432 w452 w471 w479 w509 w517 w529 w544 w563 w583 w598]
          tunnel: [w296 w321 w325 w353 w366 w390 w406 w423 w443 w461 w473 w497 w515 w529 w540 w562 w578 w599] -> w291
          tunnel: w287 -> [w309 w320 w339 w359 w375 w399 w415 w431 w451 w470 w493 w508 w521 w528 w539 w560 w565 w596]
          tunnel: [w308 w320 w339 w357 w375 w399 w415 w431 w451 w470 w493 w508 w521 w528 w539 w560 w565 w596] -> w286
          tunnel: [_ _ _ _ _ _ _ _ _ _ _ _ _ _ _ _ w576 _] -> w285
          tunnel: w283 -> [_ _ w335 _ w373 w397 w413 w429 w449 w468 w492 w506 w525 _ w538 _ w574 _]
          tunnel: w281 -> [w306 _ w323 _ _ w382 w402 w420 w438 w459 w484 _ w512 _ w537 w558 w569 w595]
          tunnel: [_ _ _ _ _ _ _ _ _ _ _ _ _ _ _ _ w572 _] -> w280
          tunnel: w278 -> [w302 w318 w337 w362 w374 w398 w414 w430 w450 w469 w480 w507 w522 w526 w530 w551 w566 w586]
          tunnel: w277 -> [w303 w319 w338 w364 w370 w394 w401 w426 w446 w465 w483 w503 w523 w527 w532 w552 w567 w587]
          tunnel: [w303 w319 w338 w363 w368 w392 w409 w424 w444 w464 w482 w501 w523 w527 w532 w552 w567 w587] -> w276
          tunnel: [w302 w318 w336 w351 w365 w389 w405 w422 w442 w460 w472 w496 w522 w526 errorcluster {"status"=FALSE, "code"=0, "source"=""} ("error out") w551 w566 w586] -> w275
          tunnel: w274 -> [_ _ _ w361 _ _ _ _ _ _ _ _ _ _ _ _ _ _]
          tunnel: w273 -> [_ _ w332 w360 _ _ _ _ _ _ _ _ _ _ _ _ _ _]
          frame "Initialize" {
            w304 = "Initial Message" ("Initial Message")
            # "#CodeNeeded - Initialize the appearance of the front panel."
            # "#CodeNeeded - Initialize your state data here."
            # "Initialize - Any operation that needs to be done before the module can receive messages. Synchronize Caller Events.vi will inform Start Module.vi that the module has launched and is ready to receive messages. Module Did Init.vi will broadcast that the module initialized."
            n121 = call "Synchronize Caller Events.vi"("error in"=w315, "Module Admin"=w306) -> ("error out"=w296:errorcluster, "Module Admin out"=w305:refnum<class "Delacor_lib_QMH_Cloneable Module Admin.lvclass">)  [unwired: 8 in]
            n122 = property on="Property Node" class="Mod Admin"(reference=w305) -> ("Accessors:Module ID"=w295:i32, "Accessors:External Launch"=w307:bool)  [unwired: 1 in, 2 out]
            n123 = Decrement(x=w295) -> (x-1=w294:i32)
            n124 = Format Into String(format string="Test Unit_%03d", w294) -> (resulting string=w292:string)  [unwired: 2 in, 1 out]
            n125 = property on="Property Node" class="VI"("Front Panel.Title"=w292) -> (reference out=w314:refnum<vi>, error out=w317:errorcluster)  [unwired: 2 in]
            n126 = Select(t=T22."Hidden" ("State"), s=w307, f=T22."Standard" ("State")) -> (s? t:f=w310:T22)
            n127 = invoke on="Invoke Node" class="VI" method="FP.Open"(reference=w314, error in=w317, "Activate"=FALSE ("Activate?"), "State"=w310) -> (reference out=w313:refnum<vi>, error out=w316:errorcluster)  [unwired: 1 in, 3 out]
            n128 = invoke on="Invoke Node" class="VI" method="FP.Center"(reference=w313, error in=w316) -> (error out=w300:errorcluster)  [unwired: 1 in, 2 out]
            n129 = Merge Errors(w300, w296) -> (w299:errorcluster)
            n130 = Bundle By Name(cluster=w309, "Status"=w304) -> (w308:T3)
            n131 = call-poly <vilib>:"Delacor_lib_QMH_Enqueue Message (poly).vi"("error in"=w299, "Message"="Binding", "Message Queue in"=w298) -> ()  [unwired: 7 in, 2 out]
            "Status" <- w304
          }
          frame "---Module Specific---" {
            # "Separator -- The following cases handle messages specific to this Module."
          }
          frame "TitleWindows" {
            n132 = Variant To Data(error in=w337, type=T9 {"Module ID"=-1, "TitleWindows"=FALSE, "dont initi"=FALSE} ("TitleWindows Argument"), Variant=w335) -> (data=w333:T9, error out=w336:errorcluster)
            n133 = Unbundle By Name(w333) -> ("TitleWindows"=w329:bool, "dont initi"=w324:bool)
            n134 = property on="Property Node" class="Mod Admin"(reference=w323) -> ("Accessors:Module ID"=w322:i32)  [unwired: 1 in, 2 out]
            n135 = call "Get Win Handle.vi"("error in (no error)"=w327, ".NET Refnum in"=w332) -> ("error out"=w328:errorcluster, "Bounds"=w330:T24, "ToInt32"=w331:i32)  [unwired: 6 in, 1 out]
            n136 = call "TileWindows.vi"("Front Panel Window:Panel Bounds"=w330, "error in (no error)"=w328, "Vertical?"=w329, "hWnd"=w331) -> ("error out"=w326:errorcluster)  [unwired: 7 in]
            n137 = case shown="True" w324 {
              tunnel: w326 -> [w342 w346]
              tunnel: [w341 w346] -> w325
              tunnel: w322 -> [w340 _]
              frame False {
                n138 = control-ref of="This VI"() -> (w343:refnum<vi>)
                n139 = call "Module Name--constant.vi"("Module ID"=w340) -> ("Module Name"=w344:string)  [unwired: 10 in]
                n140 = call "Module Did Init.vi"("This VI"=w343, "error in"=w342, "Initialized?"=TRUE, "Origin"=w344, "Module ID"=w340) -> ("error out"=w341:errorcluster)  [unwired: 6 in]
              }
              frame True {
              }
            }
          }
          frame "Binding" {
            # "Duplicate this frame when creating new messages.  Change this comment in the duplicated frame to describe this message."
            n141 = call "Set Parent(MDI).vi"("Error In"=w362, "Panel"=w360, "Number of socket"=w361, "Test Executive Manage in"=w364) -> ("Error Out"=w351:errorcluster, "UUT Result"=w347:map{i32, refnum<user-event>}, "exit"=w358:refnum<user-event>[], "Test Executive Manage out"=w363:refnum<class "Test Executive Manage.lvclass">)  [unwired: 4 in]
            n142 = Merge Errors(w355, w351) -> (w352:errorcluster)
            n143 = Bundle By Name(cluster=w359, "exit"=w358, "UUT Result"=w347) -> (w357:T3)
            n144 = call "Stall Data Flow.vim"("value in"=w352, "milliseconds to wait"=u32 10) -> ("value out"=w350:errorcluster)  [unwired: 1 out]
            n145 = call-poly <vilib>:"Delacor_lib_QMH_Enqueue Message (poly).vi"("error in"=w350, "Message Data"=T9 {"Module ID"=-1, "TitleWindows"=TRUE, "dont initi"=FALSE} ("TitleWindows Argument"), "Message"="TitleWindows", "Message Queue in"=w356) -> ("error out"=w353:errorcluster)  [unwired: 6 in, 1 out]
          }
          frame "Cofiguration" {
            # "#CodeNeeded\n1. Configure this Message Case for handling the \"Cofiguration\" message.\n2. Delete or edit this label when done."
            n146 = Variant To Data(error in=w374, type=T10 {"Module ID"=-1, "TestEngine Cofiguration"={"Break on Failure"=FALSE, "Automatically handle TestVI error"={"Enable"=FALSE, "Handle"=enum."Termination test"}, "Local Report Configuration"={"Report Folder Path"=path "", "Format"=enum."Excel", "Disable"=FALSE, "Build Date Folder?"=FALSE}, "Database Configuration"={"Connection String Expression"="", "Microsoft Data Link File"=path "", "Connection Type"=enum."Use Connection String Expression", "Enable"=FALSE}, "Ignore breakpoint"=FALSE, "Filter Result"=FALSE}} ("Cofiguration Argument"), Variant=w373) -> (data=w371:T10, error out=w369:errorcluster)
            n147 = Unbundle By Name(w371) -> ("TestEngine Cofiguration"=w367:T11)  [unwired: 1 out]
            n148 = call <vilib>:"Test Engine Configuration.vi"("error in (no error)"=w369, "TestEngine Cofiguration"=w367, "Test Executive Manage in"=w370) -> ("error out"=w365:errorcluster, "Test Executive Manage out"=w368:refnum<class "Test Executive Manage.lvclass">)  [unwired: 7 in]
            n149 = Merge Errors(w376, w365) -> (w366:errorcluster)
          }
          frame "Load Sequence" {
            # "#CodeNeeded\n1. Configure this Message Case for handling the \"Load Sequence\" message.\n2. Delete or edit this label when done."
            n150 = property on="Property Node" class="Mod Admin"(reference=w382) -> ("Accessors:Module ID"=w381:i32)  [unwired: 1 in, 2 out]
            n151 = Variant To Data(error in=w398, type=T15 {"Module ID"=-1, "File Pathname"=path "", "Sequence"="Main_Sequence"} ("Load Sequence Argument"), Variant=w397) -> (data=w395:T15, error out=w393:errorcluster)
            n152 = Unbundle By Name(w395) -> ("File Pathname"=w379:path, "Sequence"=w391:string)
            n153 = Path to Array of Strings(0:w379) -> (2:w385:string[])  [unwired: 1 out]
            n154 = Reverse 1D Array(array=w385) -> (reversed array=w384:string[])
            n155 = Index Array(array=w384) -> (element #1=w377:string, element #2=w383:string)  [unwired: 2 in]
            n156 = Format Into String(format string="Load Sequence %s", w377) -> (resulting string=w378:string)  [unwired: 2 in, 1 out]
            n157 = call <vilib>:"Load Sequence.vi"("error in (no error)"=w393, "Sequence"=w391, "File Pathname"=w379, "Test Executive Manage in"=w394) -> ("error out"=w389:errorcluster, "Test Executive Manage out"=w392:refnum<class "Test Executive Manage.lvclass">)  [unwired: 6 in]
            n158 = call "Status Updated.vi"("Status"=w378, "Module ID"=w381) -> ()  [unwired: 9 in, 1 out]
            n159 = property on="Property Node" class="VI"() -> ("Front Panel.Title"=w387:string)  [unwired: 2 in, 2 out]
            n160 = Merge Errors(w400, w389) -> (w390:errorcluster)
            n161 = Format Into String(format string="%s (../%s/%s)", w387, w383, w377) -> (resulting string=w386:string)  [unwired: 2 in, 1 out]
            n162 = property on="Property Node" class="VI"("Front Panel.Title"=w386) -> ()  [unwired: 2 in, 2 out]
          }
          frame "Write SN" {
            # "#CodeNeeded\n1. Configure this Message Case for handling the \"Write SN\" message.\n2. Delete or edit this label when done."
            n163 = Variant To Data(error in=w414, type=T16 {"Module ID"=-1, "Socket"=0, "Serial Number"=""} ("Write SN Argument"), Variant=w413) -> (data=w411:T16, error out=w410:errorcluster)
            n164 = property on="Property Node" class="Mod Admin"(reference=w402) -> ("Accessors:Module ID"=w403:i32)  [unwired: 1 in, 2 out]
            n165 = Unbundle By Name(w411) -> ("Socket"=w408:i32, "Serial Number"=w407:string)
            n166 = call "Status Updated.vi"("Status"="Write SN" ("format string"), "Module ID"=w403) -> ()  [unwired: 9 in, 1 out]
            n167 = call <vilib>:"Set UUT Serial Number.vi"("error in (no error)"=w410, "Serial Number"=w407, "Socket"=w408, "Test Executive Manage in"=w401) -> ("error out"=w405:errorcluster, "Test Executive Manage out"=w409:refnum<class "Test Executive Manage.lvclass">)  [unwired: 6 in]
            n168 = Merge Errors(w416, w405) -> (w406:errorcluster)
          }
          frame "UUT Test" {
            # "#CodeNeeded\n1. Configure this Message Case for handling the \"UUT Test\" message.\n2. Delete or edit this label when done."
            n169 = Variant To Data(error in=w430, type=T17 {"Module ID"=-1, "Socket"=0} ("UUT Test Argument"), Variant=w429) -> (data=w427:T17, error out=w425:errorcluster)
            n170 = property on="Property Node" class="Mod Admin"(reference=w420) -> ("Accessors:Module ID"=w421:i32)  [unwired: 1 in, 2 out]
            n171 = Unbundle By Name(w427) -> ("Socket"=w418:i32)  [unwired: 1 out]
            n172 = Format Into String(format string="Socket%d Start Test", w418) -> (resulting string=w417:string)  [unwired: 2 in, 1 out]
            n173 = call "Status Updated.vi"("Status"=w417, "Module ID"=w421) -> ()  [unwired: 9 in, 1 out]
            n174 = call <vilib>:"UUT Test.vi"("error in (no error)"=w425, "Socket"=w418, "Test Executive Manage in"=w426) -> ("error out"=w422:errorcluster, "Test Executive Manage out"=w424:refnum<class "Test Executive Manage.lvclass">)  [unwired: 7 in]
            n175 = Merge Errors(w432, w422) -> (w423:errorcluster)
          }
          frame "UUTs Test" {
            # "#CodeNeeded\n1. Configure this Message Case for handling the \"UUTs Test\" message.\n2. Delete or edit this label when done."
            n176 = Variant To Data(error in=w450, type=T18 {"Module ID"=-1, "Enable Socket"=[]} ("UUTs Test Argument"), Variant=w449) -> (data=w447:T18, error out=w445:errorcluster)
            n177 = property on="Property Node" class="Mod Admin"(reference=w438) -> ("Accessors:Module ID"=w441:i32)  [unwired: 1 in, 2 out]
            n178 = Unbundle By Name(w447) -> ("Enable Socket"=w437:bool[])  [unwired: 1 out]
            n179 = for {
              tunnel: w437 -> [w456] mode=indexing
              tunnel: [w453] -> w436 mode=indexing
              n180 = Select(t="T", s=w456, f="F") -> (s? t:f=w453:string)
            }
            n181 = Array To Spreadsheet String(delimiter (Tab)=",", array=w436, 3:"%s" ("format string")) -> (spreadsheet string=w433:string)
            n182 = call <vilib>:"UUTs Test.vi"("error in (no error)"=w445, "Enable Socket"=w437, "Test Executive Manage in"=w446) -> ("error out"=w442:errorcluster, "Test Executive Manage out"=w444:refnum<class "Test Executive Manage.lvclass">)  [unwired: 7 in]
            n183 = Format Into String(format string="Socket%s Start Test", w433) -> (resulting string=w439:string)  [unwired: 2 in, 1 out]
            n184 = Merge Errors(w452, w442) -> (w443:errorcluster)
            n185 = call "Status Updated.vi"("Status"=w439, "Module ID"=w441) -> ()  [unwired: 9 in, 1 out]
          }
          frame "Terminate Test" {
            n186 = Variant To Data(error in=w469, type=T19 {"Module ID"=-1, "Abort VI"=FALSE} ("Terminate Test Argument"), Variant=w468) -> (data=w466:T19, error out=w463:errorcluster)
            n187 = property on="Property Node" class="Mod Admin"(reference=w459) -> ("Accessors:Module ID"=w458:i32)  [unwired: 1 in, 2 out]
            n188 = Unbundle By Name(w466) -> ("Abort VI"=w462:bool)
            n189 = call "Status Updated.vi"("Status"="Terminate All", "Module ID"=w458) -> ()  [unwired: 9 in, 1 out]
            n190 = call <vilib>:"Terminate All Test.vi"("Abort VI"=w462, "error in (no error)"=w463, "Test Executive Manage in"=w465) -> ("error out"=w460:errorcluster, "Test Executive Manage out"=w464:refnum<class "Test Executive Manage.lvclass">)  [unwired: 7 in]
            n191 = Merge Errors(w471, w460) -> (w461:errorcluster)
          }
          frame "Get Variable" {
            n192 = property class="Mod Admin"(reference=w484) -> ("Accessors:Module ID"=w485:i32)  [unwired: 1 in, 2 out]
            n193 = Variant To Data(error in=w479, type=T21 {"Module ID"=-1, "Socket"=0, "Variable"="", "Wait Notifier"=refnum, "wait for reply"=FALSE} ("Get Variable Argument"), Variant=w492) -> (data=w490:T21, error out=w478:errorcluster)
            n194 = Unbundle By Name(w490) -> ("Socket"=w481:i32, "Variable"=w477:string, "Wait Notifier"=w489:refnum<notifier>, "wait for reply"=w488:bool)
            n195 = call <vilib>:"Get Variable.vi"("Socket"=w481, "error in (no error)"=w480, "Variable"=w477, "Test Executive Manage in"=w483) -> ("error out"=w472:errorcluster, "Variable not found?"=w475:bool, "Value"=w476:variant, "Test Executive Manage out"=w482:refnum<class "Test Executive Manage.lvclass">, "timed out?"=w474:bool)  [unwired: 3 in]
            n196 = Bundle By Name(cluster=T23 {"Module ID"=-1, "Value"=variant, "Variable not found?"=FALSE, "timed out?"=FALSE, "error"={"status"=FALSE, "code"=0, "source"=""}} ("Get Variable (Reply Payload)"), "Module ID"=w485, "Value"=w476, "Variable not found?"=w475, "timed out?"=w474, "error"=w472) -> (w487:T23)
            n197 = Merge Errors(w478, w472) -> (w473:errorcluster)
            n198 = case "DQMH_FIRE_NOTIFIER" shown="False" w488 {
              tunnel: w489 -> [_ w495]
              tunnel: w487 -> [_ w494]
              frame False {
              }
              frame True {
                n199 = Send Notification(notification=w494, notifier=w495) -> ()  [unwired: 1 in, 2 out]
              }
            }
          }
          frame "Set Variable" {
            # "#CodeNeeded\n1. Configure this Message Case for handling the \"Set Variable\" message.\n2. Delete or edit this label when done."
            n200 = Variant To Data(error in=w507, type=T20 {"Module ID"=-1, "Variable"="", "Socket"=0, "Value"=variant} ("Set Variable Argument"), Variant=w506) -> (data=w504:T20, error out=w502:errorcluster)
            n201 = Unbundle By Name(w504) -> ("Socket"=w498:i32, "Variable"=w500:string, "Value"=w499:variant)
            n202 = call <vilib>:"Set Variable.vi"("Socket"=w498, "error in (no error)"=w502, "Value"=w499, "Variable"=w500, "Test Executive Manage in"=w503) -> ("error out"=w496:errorcluster, "Test Executive Manage out"=w501:refnum<class "Test Executive Manage.lvclass">)  [unwired: 5 in]
            n203 = Merge Errors(w509, w496) -> (w497:errorcluster)
          }
          frame "Get UUT Result" {
            n204 = Variant To Data(type=T4 {"Station"=0, "Socket"=0, "DetailTestResult"=[], "Report Path"=path "", "General"={"Sequence Path"=path "", "Serial Number"="", "Test Date Time"=timestamp(0 s since 1904-01-01), "UUT Status"="", "Faulty Item"="", "Seconds Executing"=0.0}} ("output cluster"), Variant=w525) -> (data=w513:T4, error out=w514:errorcluster)  [unwired: 1 in]
            n205 = Unbundle By Name(w513) -> ("Socket"=w519:i32)
            n206 = Unbundle By Name(w521) -> ("UUT Result"=w520:map{i32, refnum<user-event>})
            n207 = Look In Map(map=w520, key=w519) -> (value=w518:refnum<user-event>)  [unwired: 1 in, 1 out]
            n208 = property class="Mod Admin"(reference=w512) -> ("Accessors:Module ID"=w511:i32)  [unwired: 1 in, 2 out]
            n209 = Generate User Event(user event=w518, event data cluster=w513, error in=w517) -> (error out=w516:errorcluster)  [unwired: 1 in, 1 out]
            n210 = call "Send UUT Result.vi"("Station"=w511, "UUT Result"=w513) -> ()  [unwired: 9 in, 1 out]
            n211 = Merge Errors(w516, w514) -> (w515:errorcluster)
            n212 = call "Status Updated.vi"("Status"="Test completed", "Module ID"=w511) -> ()  [unwired: 9 in, 1 out]
          }
          frame "---Exit and Error Handling---" {
            # "Separator - the following cases handle errors and exit messages."
          }
          frame "Error" {
            # "#CodeRecommended - If the module is running in standalone mode (External Launch = FALSE), this code will pop up an error dialog and call the 'Exit' message if an error occurs. Add more fine-grained error management here."
            # "Error - Check the error message data and respond accordingly. This message is sent by the \"Error Handler\" VIs at the end of each loop in this application."
            n213 = property on="Property Node" class="Mod Admin"(reference=w537) -> ("Accessors:External Launch"=w536:bool, "Accessors:Module ID"=w534:i32)  [unwired: 1 in, 2 out]
            n214 = Variant To Data(error in=w544, type=errorcluster {"status"=FALSE, "code"=0, "source"=""} ("error constant"), Variant=w538) -> (data=w533:errorcluster, error out=w542:errorcluster)
            n215 = local write "error out"(w533) -> ()
            n216 = call <vilib>:"Simple Error Handler.vi"("error in (no error)"=w530) -> ()  [unwired: 4 in, 5 out]
            n217 = call "Error Reported.vi"("Error"=w533, "Module ID"=w534) -> ()  [unwired: 9 in, 1 out]
            n218 = case shown="False" w536 {
              tunnel: [w549 _] -> w541
              tunnel: w535 -> [w547 _]
              tunnel: w533 -> [w548 _]
              frame False {
                n219 = disable-structure shown="Default" {
                  disable-tunnel: w548 -> [w550 _]
                  frame condition #0 (active) {
                    # "If the module is running standalone, then pop up an error dialog and call the \"Exit\" message."
                    n220 = call <vilib>:"Simple Error Handler.vi"("error in (no error)"=w550) -> ()  [unwired: 4 in, 5 out]
                  }
                  frame condition #1 {
                    # "To prevent the Simple Error Handler VI from being loaded (e.g. when deploying to a Real-Time target), add the Conditional Disable Symbol \"DQMH_Disable_SEH\" to your project and set it to TRUE."
                  }
                }
                n221 = call-poly <vilib>:"Delacor_lib_QMH_Enqueue Message (poly).vi"("Priority Message? (F)"=TRUE, "Message"="Exit", "Message Queue in"=w547) -> ("error out"=w549:errorcluster)  [unwired: 7 in, 1 out]
              }
              frame True {
                # "If the module was launched externally, calling the Error Reported broadcast VI is the only action performed by the \"Error\" message. The module's caller can then process the error appropriately."
              }
            }
            n222 = Merge Errors(w542, w541) -> (w540:errorcluster)
          }
          frame "Simulate MHL Error" {
            # "#DQMH_HowTo The 'Simulate MHL Error' button  illustrates how the MHL handles errors. This event is instructional in nature and can be removed."
            # "Simulate an error occurring at the MHL"
            n223 = property on="Property Node" class="Mod Admin"(reference=w558) -> ("Accessors:Module ID"=w559:i32)  [unwired: 1 in, 2 out]
            n224 = call "Module Name--constant.vi"("Module ID"=w559) -> ("Module Name"=w554:string)  [unwired: 10 in]
            n225 = Format Into String(format string="Simulated error originating at Message Handling Loop in %s", w554) -> (resulting string=w555:string)  [unwired: 2 in, 1 out]
            n226 = call <vilib>:"Error Cluster From Error Code.vi"("show call chain? (False)"=TRUE, "error message (\"\")"=w555, "error code (0)"=5001) -> ("error out"=w561:errorcluster)  [unwired: 6 in]
            n227 = Merge Errors(w563, w561) -> (w562:errorcluster)
          }
          frame "Exit" {
            w575 = 91  # 91: not all Exit messages will have an argument
            w576 = TRUE  # Stop the VI
            # "Release the message queue reference"
            # "#CodeNeeded - Add any required cleanup code here."
            # "Exit - Exit the application."
            n228 = Variant To Data(error in=w583, type=T8 {"Module ID"=-1, "Origin"="", "Exit via Stop Module Req?"=FALSE, "Wait for Module to stop?"=FALSE} ("Stop Argument"), Variant=w574) -> (data=w571:T8, error out=w579:errorcluster)
            n229 = call <vilib>:"Clear Errors.vi"("error in (no error)"=w579, "specific error code to clear (0: all)"=w575) -> ("error out"=w582:errorcluster)  [unwired: 4 in, 1 out]
            n230 = property on="Property Node" class="Mod Admin"(reference=w569) -> ("Accessors:Module ID"=w568:i32)  [unwired: 1 in, 2 out]
            n231 = control-ref of="This VI"() -> (w570:refnum<vi>)
            n232 = call-dynamic "Delacor_lib_QMH_Release Message Queue.vi"("error in"=w582, "Message Queue"=w577) -> ("error out"=w581:errorcluster)  [unwired: 9 in]
            n233 = call "Handle Exit.vi"("Stop Argument"=w571, "Module Admin in"=w569, "VI reference"=w570) -> ("error out"=w580:errorcluster, "Wait for Stop?"=w572:bool)  [unwired: 7 in]
            n234 = Merge Errors(w581, w580) -> (w578:errorcluster)
            n235 = Unbundle By Name(w565) -> ("exit"=w564:refnum<user-event>[])
            n236 = call "Error Reported.vi"("Error"=w578, "Module ID"=w568) -> ()  [unwired: 9 in, 1 out]
            n237 = for {
              tunnel: w564 -> [w584] mode=indexing
              n238 = Generate User Event(user event=w584, event data cluster=TRUE ("event data")) -> ()  [unwired: 2 in, 2 out]
            }
          }
          frame Default {
            # "'Default' case only runs if there is a message that isn't defined in any of the other cases.  Output a programming error."
            n239 = property on="Property Node" class="Mod Admin"(reference=w595) -> ("Accessors:Module ID"=w594:i32)  [unwired: 1 in, 2 out]
            n240 = call "Module Name--constant.vi"("Module ID"=w594) -> ("Module Name"=w588:string)  [unwired: 10 in]
            n241 = Format Into String(format string="The invalid message string \"%s\" was received in the Message Handling Loop for module \"%s\".", w589, w588) -> (resulting string=w591:string)  [unwired: 2 in, 1 out]
            n242 = call <vilib>:"Error Cluster From Error Code.vi"("show call chain? (False)"=TRUE, "error message (\"\")"=w591, "error code (0)"=1) -> ("error out"=w597:errorcluster)  [unwired: 6 in]
            n243 = Merge Errors(w598, w597) -> (w599:errorcluster)
          }
        }
        n244 = call-dynamic "Delacor_lib_QMH_Error Handler - Message Handling Loop.vi"("error in"=w291, "Message Queue in"=w282) -> ("dup error in"=w288:errorcluster)  [unwired: 8 in, 1 out]
      }
    }
    frame Error {
      n245 = call "Synchronize Caller Events.vi"("Module Admin"=w605) -> ("Module Admin out"=w604:refnum<class "Delacor_lib_QMH_Cloneable Module Admin.lvclass">)  [unwired: 9 in, 1 out]
      n246 = property on="Property Node" class="Mod Admin"(reference=w604) -> ("Accessors:Module ID"=w603:i32)  [unwired: 1 in, 2 out]
      n247 = call-dynamic "Delacor_lib_QMH_Release Message Queue.vi"("error in"=w611, "Message Queue"=w602) -> ("error out"=w610:errorcluster)  [unwired: 9 in]
      n248 = call "Module Name--constant.vi"("Module ID"=w603) -> ("Module Name"=w608:string)  [unwired: 10 in]
      n249 = Format Into String(format string="An error occurred during initialization. %s is no longer running.", w608) -> (resulting string=w606:string)  [unwired: 2 in, 1 out]
      n250 = call "Error Reported.vi"("Additional Information"=w606, "Error"=w610, "Module ID"=w603) -> ()  [unwired: 8 in, 1 out]
    }
  }
  n251 = Merge Errors(w31, w30) -> (w32:errorcluster)
  n252 = call "Close Module.vi"("error in"=w32, "Wait for stop?"=w21, "Module Admin in"=w17) -> ("error out"=w2:errorcluster, "External Launch"=w20:bool, "Module Admin out"=w22:refnum<class "Delacor_lib_QMH_Cloneable Module Admin.lvclass">)  [unwired: 6 in]
  n253 = call <vilib>:"Stop Engine.vi"("error in (no error)"=w12, "Test Executive Manage in"=w13) -> ("error out"=w11:errorcluster)  [unwired: 9 in]
  n254 = Unregister For Events(event registration refnum=w26, error in=w2) -> (error out=w1:errorcluster)
  n255 = Merge Errors(w2, w11) -> (w8:errorcluster)
  n256 = call <vilib>:"Clear Errors.vi"("error in (no error)"=w1) -> ()  [unwired: 5 in, 2 out]
  n257 = case "External Launch?" shown="True" w20 {
    tunnel: w8 -> [_ w612]
    frame False {
    }
    frame True {
      n258 = case shown="Error" w612 {
        frame No Error {
          n259 = invoke class="VI" method="FP.Close"() -> ()  [unwired: 3 in, 3 out]
        }
        frame Error {
          n260 = invoke class="VI" method="FP.Open"("Activate"=TRUE ("Activate?")) -> ()  [unwired: 4 in, 5 out]
        }
      }
    }
  }
  n261 = call <vilib>:"Simple Error Handler.vi"("error in (no error)"=w8) -> ("error out"=→"error out":errorcluster)  [unwired: 4 in, 4 out]
  n262 = local write "Module Admin"(w22) -> ()
